vi "Create from SSH.vi"(8 "Error In":errorcluster, 11 "SSH":refnum<class "SSH.lvclass">) -> (0 "Error Out":errorcluster, 3 "Known Host":refnum<class "Known Host.lvclass">)   [LabVIEW 2021, in "Field_RnD_Services_LIBSSH2_Toolkit.lvlib" / "Known Host.lvclass"]
doc: "Creates a new Known Host object from a SSH context."
uses:
  Known Host.lvclass
  SSH/SSH.lvclass
  Known Host.lvclass/Known Host.ctl
  Field_RnD_Services_LIBSSH2_Toolkit.lvlib
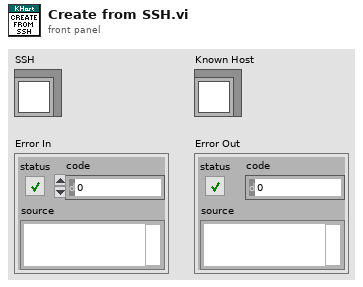
[diagram p1: front panel]
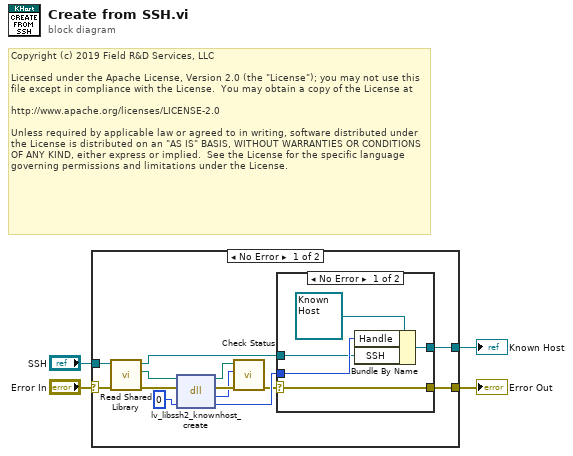
[diagram p0: block diagram]
diagram:
  # "Copyright (c) 2019 Field R&D Services, LLC\n\nLicensed under the Apache License, Version 2.0 (the \"License\"); you may not use this file except in compliance with the License.  You may obtain a copy of the License at\n\nhttp://www.apache.org/licenses/LICENSE-2.0\n\nUnless required by applicable law or agreed to in writing, software distributed under the License is distributed on an \"AS IS\" BASIS, WITHOUT WARRANTIES OR CONDITIONS OF ANY KIND, either express or implied.  See the License for the specific language governing permissions and limitations under the License."
  n1 = case shown="No Error" "Error In" {
    selector: "Error In" -> [w8 w24]
    tunnel: [w10 w24] -> w3
    tunnel: [w17 _] -> w2
    tunnel: "SSH" -> [w9 _]
    frame No Error {
      n2 = call "Read Shared Library.vi"("Error In"=w8, "SSH In"=w9) -> ("Error Out"=w7:errorcluster, "libssh2lv Shared Library"=w6:path, "SSH Out"=w5:refnum<class "SSH.lvclass">)  [unwired: 7 in]
      n3 = dll-call lib="D:/Users/cfield/Code/Field R&D Services/SSH/LV-LIBSSH2/LabVIEW/trunk/src/Toolkit/Support/lv-libssh2.*" fn="lv_libssh2_knownhost_create"(path in=w6, error in=w7, "handle"=u64 0) -> (path out=w13:path, error out=w14:errorcluster, "status"=w12:i32, "handle"=w15:u64)  [unwired: 1 in]
      n4 = call "Check Status.vi"("Error In"=w14, "Status"=w12, "libssh2lv Shared Library In"=w13) -> ("Error Out"=w11:errorcluster)  [unwired: 7 in, 1 out]
      n5 = case shown="No Error" w11 {
        selector: w11 -> [w20 w23]
        tunnel: [w22 _] -> w17
        tunnel: w15 -> [w21 _]
        tunnel: [w20 w23] -> w10
        tunnel: w5 -> [w18 _]
        frame No Error {
          n6 = Bundle By Name(cluster=refnum<class "Known Host.lvclass"> refnum ("Toolkit.lvlib:KnownHost.lvclass"), "Handle"=w21, "SSH"=w18) -> (w22:refnum<class "Known Host.lvclass">)
        }
        frame Error {
        }
      }
    }
    frame Error {
    }
  }
  "Error Out" <- w3
  "Known Host" <- w2
